vi "Parse Heatup Test Data.vi"(4 "34970 Data Raw":string[](array[string]), 5 "MW100 Data Raw":string[](array[string]), 6 "Agilent Read All?":bool=TRUE, 7 "Agilent Label Array":string[](array[string]), 8 "Serial Data":string="0:0:0 UE 36 LE 0 COMP 0 FAN1 0 FAN2 0 SP:0 0 0 0 0 0 C030", 9 "34970 Data":string[](array[string]), 10 "Power Data":string[](array[string]), 11 "MW100 Data":string[](array[string])) -> (2 "Output Data":string[][](array[string]))   [LabVIEW 2012]
uses:
  Global HEWH.vi
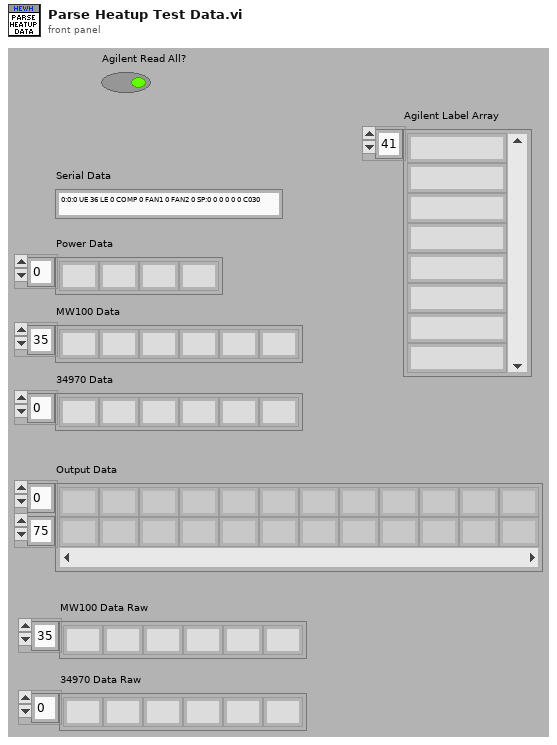
[diagram p1: front panel]
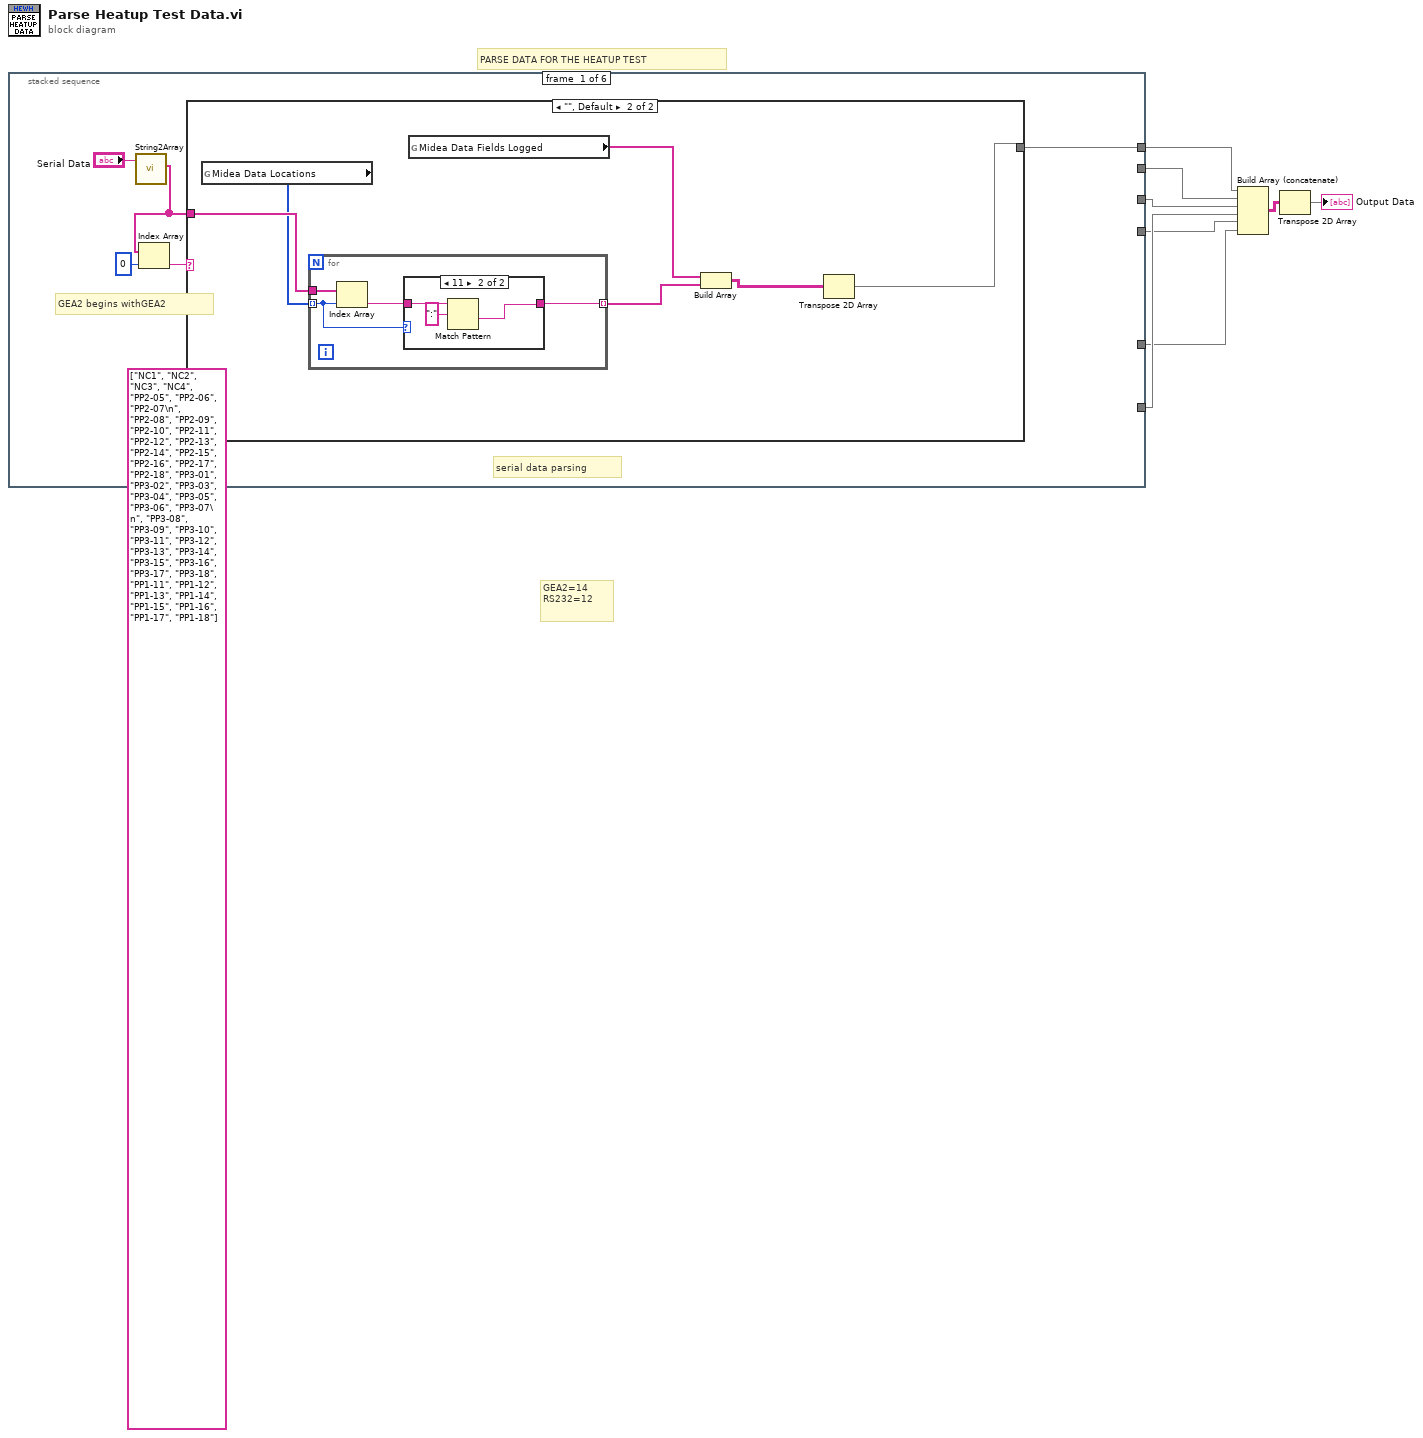
[diagram p0: block diagram]
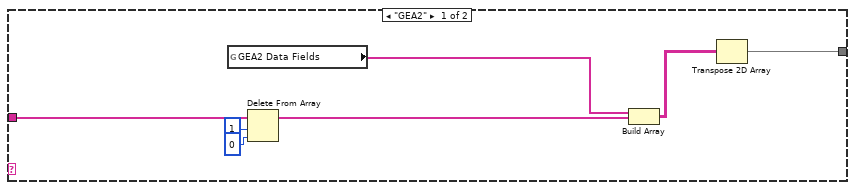
[diagram p2: hidden frame]
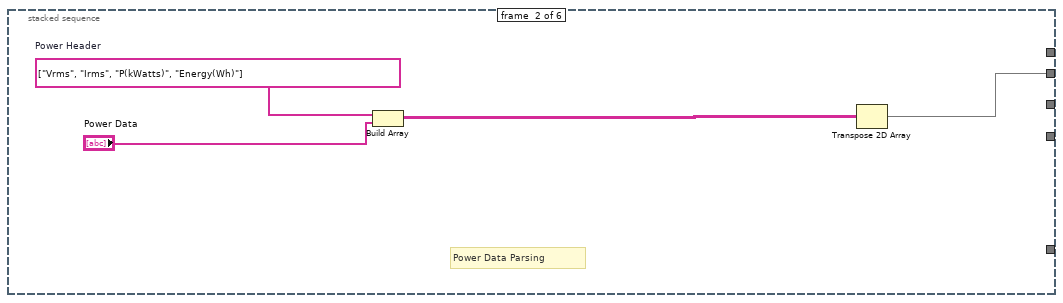
[diagram p4: hidden frame]
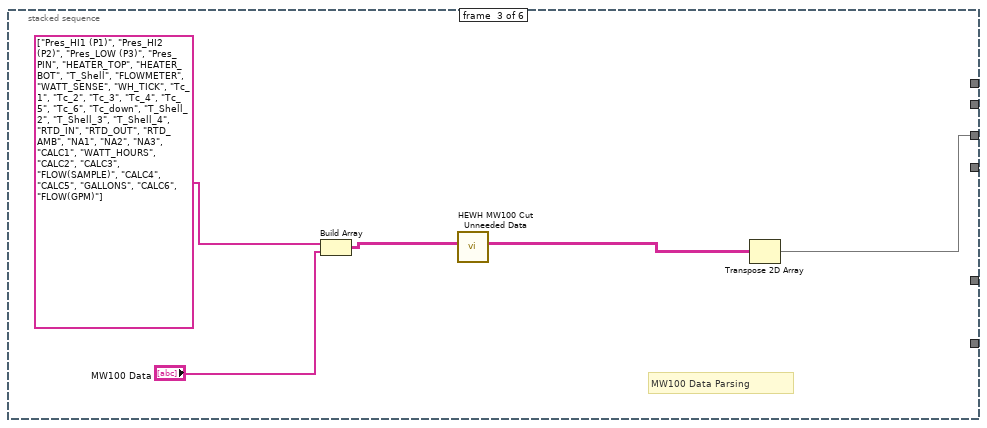
[diagram p5: hidden frame]
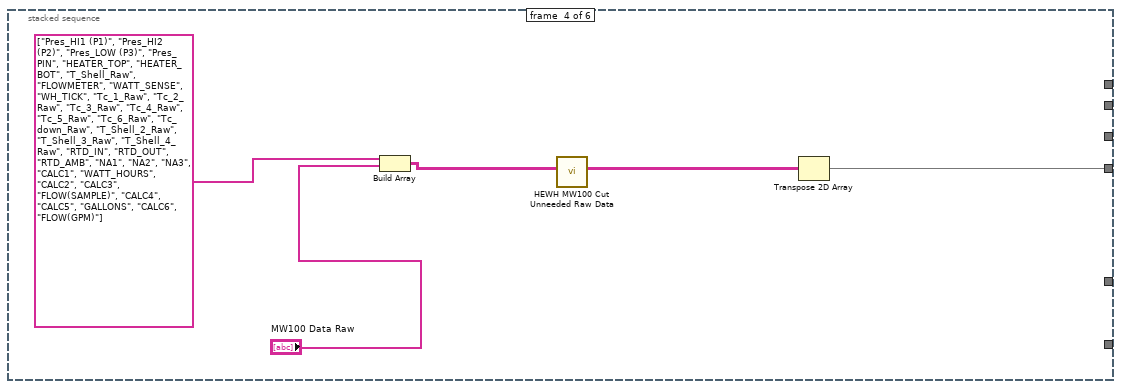
[diagram p6: hidden frame]
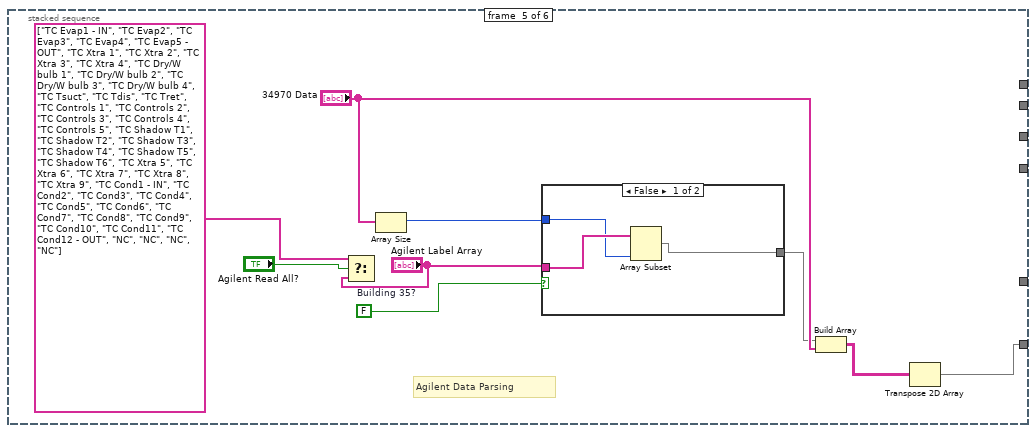
[diagram p7: hidden frame]
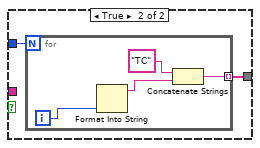
[diagram p8: hidden frame]
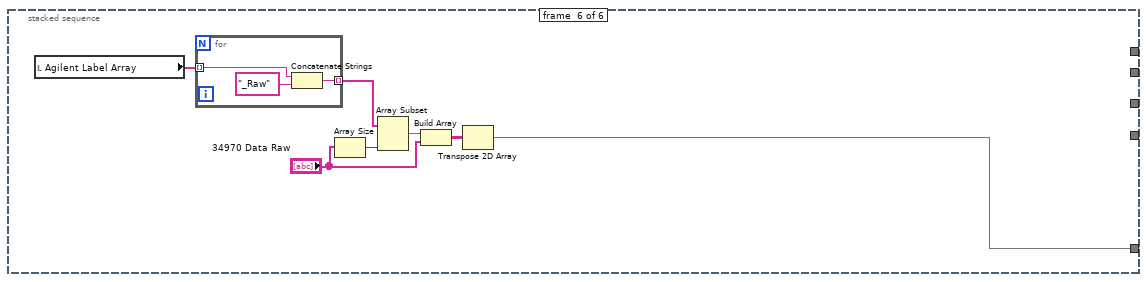
[diagram p9: hidden frame]
diagram:
  (unwired) string[] ["NC1", "NC2", "NC3", "NC4", "PP2-05", "PP2-06", "PP2-07\n", "PP2-08", "PP2-09", "PP2-10", "PP2-11", "PP2-12", "PP2-13", "PP2-14", "PP2-15", "PP2-16", "PP2-17", "PP2-18", "PP3-01", "PP3-02", "PP3-03", "PP3-04", "PP3-05", "PP3-06", "PP3-07\n", "PP3-08", "PP3-09", "PP3-10", "PP3-11", "PP3-12", "PP3-13", "PP3-14", "PP3-15", "PP3-16", "PP3-17", "PP3-18", "PP1-11", "PP1-12", "PP1-13", "PP1-14", "PP1-15", "PP1-16", "PP1-17", "PP1-18"] ("appended array")
  # "GEA2=14\nRS232=12"
  # "PARSE DATA FOR THE HEATUP TEST"
  n1 = stacked-sequence {
    tunnel: [w9 _ _ _ _ _] -> w7
    tunnel: [_ w35 _ _ _ _] -> w6
    tunnel: [_ _ w41 _ _ _] -> w4
    tunnel: [_ _ _ _ w50 _] -> w3
    tunnel: [_ _ _ w44 _ _] -> w2
    tunnel: [_ _ _ _ _ w67] -> w1
    frame #0 {
      # "GEA2 begins withGEA2"
      # "serial data parsing"
      n2 = call "String2Array.vi"("String"="Serial Data") -> ("Array"=w10:string[])  [unwired: 10 in]
      n3 = Index Array(array=w10, index=0) -> (element=w11:string)
      n4 = case shown="\"\", Default" w11 {
        tunnel: w10 -> [w18 w26]
        tunnel: [w19 w23] -> w9
        frame "GEA2" {
          n5 = global read "Global HEWH.vi" "GEA2 Data Fields"() -> (w14:string[])
          n6 = Delete From Array(array=w18, length=1, index=0) -> (array with subset deleted=w15:string[])  [unwired: 1 out]
          n7 = Build Array(w14, w15) -> (w20:string[][])
          n8 = Transpose 2D Array(2D array=w20) -> (transposed array=w19:string[][])
        }
        frame "", Default {
          n9 = global read "Global HEWH.vi" "Midea Data Locations"() -> (w21:i32[])
          n10 = for {
            tunnel: w26 -> [w30]
            tunnel: w21 -> [w29] mode=indexing
            tunnel: [w27] -> w25 mode=indexing
            n11 = Index Array(array=w30, index=w29) -> (element=w28:string)
            n12 = case shown="11" w29 {
              tunnel: w28 -> [w31 w34]
              tunnel: [w31 w32] -> w27
              frame 0, Default {
              }
              frame 11 {
                n13 = Match Pattern(string=w34, regular expression=":") -> (after substring=w32:string)  [unwired: 1 in, 3 out]
              }
            }
          }
          n14 = global read "Global HEWH.vi" "Midea Data Fields Logged"() -> (w22:string[])
          n15 = Build Array(w22, w25) -> (w24:string[][])
          n16 = Transpose 2D Array(2D array=w24) -> (transposed array=w23:string[][])
        }
      }
    }
    frame #1 {
      w36 = string[] ["Vrms", "Irms", "P(kWatts)", "Energy(Wh)"]  # Power Header
      # "Power Data Parsing"
      n17 = Build Array(w36, "Power Data") -> (w38:string[][])
      n18 = Transpose 2D Array(2D array=w38) -> (transposed array=w35:string[][])
    }
    frame #2 {
      # "MW100 Data Parsing"
      n19 = Build Array(string[] ["Pres_HI1 (P1)", "Pres_HI2 (P2)", "Pres_LOW (P3)", "Pres_PIN", "HEATER_TOP", "HEATER_BOT", "T_Shell", "FLOWMETER", "WATT_SENSE", "WH_TICK", "Tc_1", "Tc_2", "Tc_3", "Tc_4", "Tc_5", "Tc_6", "Tc_down", "T_Shell_2", "T_Shell_3", "T_Shell_4", "RTD_IN", "RTD_OUT", "RTD_AMB", "NA1", "NA2", "NA3", "CALC1", "WATT_HOURS", "CALC2", "CALC3", "FLOW(SAMPLE)", "CALC4", "CALC5", "GALLONS", "CALC6", "FLOW(GPM)"] ("output array"), "MW100 Data") -> (w40:string[][])
      n20 = call "HEWH MW100 Cut Unneeded Data.vi"("MW100 Data In"=w40) -> ("MW100 Data Out"=w39:string[][])  [unwired: 10 in]
      n21 = Transpose 2D Array(2D array=w39) -> (transposed array=w41:string[][])
    }
    frame #3 {
      n22 = Build Array(string[] ["Pres_HI1 (P1)", "Pres_HI2 (P2)", "Pres_LOW (P3)", "Pres_PIN", "HEATER_TOP", "HEATER_BOT", "T_Shell_Raw", "FLOWMETER", "WATT_SENSE", "WH_TICK", "Tc_1_Raw", "Tc_2_Raw", "Tc_3_Raw", "Tc_4_Raw", "Tc_5_Raw", "Tc_6_Raw", "Tc_down_Raw", "T_Shell_2_Raw", "T_Shell_3_Raw", "T_Shell_4_Raw", "RTD_IN", "RTD_OUT", "RTD_AMB", "NA1", "NA2", "NA3", "CALC1", "WATT_HOURS", "CALC2", "CALC3", "FLOW(SAMPLE)", "CALC4", "CALC5", "GALLONS", "CALC6", "FLOW(GPM)"] ("output array"), "MW100 Data Raw") -> (w46:string[][])
      n23 = call "HEWH MW100 Cut Unneeded Raw Data.vi"("MW100 Data In"=w46) -> ("MW100 Data Out"=w45:string[][])  [unwired: 10 in]
      n24 = Transpose 2D Array(2D array=w45) -> (transposed array=w44:string[][])
    }
    frame #4 {
      w56 = FALSE  # Building 35?
      # "Agilent Data Parsing"
      n25 = Select(t=string[] ["TC Evap1 - IN", "TC Evap2", "TC Evap3", "TC Evap4", "TC Evap5 - OUT", "TC Xtra 1", "TC Xtra 2", "TC Xtra 3", "TC Xtra 4", "TC Dry/W bulb 1", "TC Dry/W bulb 2", "TC Dry/W bulb 3", "TC Dry/W bulb 4", "TC Tsuct", "TC Tdis", "TC Tret", "TC Controls 1", "TC Controls 2", "TC Controls 3", "TC Controls 4", "TC Controls 5", "TC Shadow T1", "TC Shadow T2", "TC Shadow T3", "TC Shadow T4", "TC Shadow T5", "TC Shadow T6", "TC Xtra 5", "TC Xtra 6", "TC Xtra 7", "TC Xtra 8", "TC Xtra 9", "TC Cond1 - IN", "TC Cond2", "TC Cond3", "TC Cond4", "TC Cond5", "TC Cond6", "TC Cond7", "TC Cond8", "TC Cond9", "TC Cond10", "TC Cond11", "TC Cond12 - OUT", "NC", "NC", "NC", "NC"] ("output array"), s="Agilent Read All?", f="Agilent Label Array") -> ()  [unwired: 1 out]
      n26 = Array Size(array="34970 Data") -> (size(s)=w55:i32)
      n27 = case shown="False" w56 {
        tunnel: w55 -> [w59 w62]
        tunnel: [w58 w61] -> w53
        tunnel: "Agilent Label Array" -> [w60 _]
        frame False {
          n28 = Array Subset(array=w60, length=w59) -> (w58:string[])  [unwired: 1 in]
        }
        frame True {
          n29 = for {
            N: w62 -> [_]
            tunnel: [w63] -> w61 mode=indexing
            i -> [w66]
            n30 = Format Into String(w66) -> (resulting string=w65:string)  [unwired: 3 in, 1 out]
            n31 = Concatenate Strings("TC" ("string"), w65) -> (w63:string)
          }
        }
      }
      n32 = Build Array(w53, "34970 Data") -> (w51:string[][])
      n33 = Transpose 2D Array(2D array=w51) -> (transposed array=w50:string[][])
    }
    frame #5 {
      n34 = local read "Agilent Label Array"() -> (w69:string[])
      n35 = for {
        tunnel: w69 -> [w76] mode=indexing
        tunnel: [w74] -> w68 mode=indexing
        n36 = Concatenate Strings(w76, "_Raw" ("string")) -> (w74:string)
      }
      n37 = Array Size(array="34970 Data Raw") -> (size(s)=w73:i32)
      n38 = Array Subset(array=w68, length=w73) -> (w72:string[])  [unwired: 1 in]
      n39 = Build Array(w72, "34970 Data Raw") -> (w70:string[][])
      n40 = Transpose 2D Array(2D array=w70) -> (transposed array=w67:string[][])
    }
  }
  n41 = Build Array (concatenate)(w7, w6, w4, w3, w2, w1) -> (w8:string[][])
  n42 = Transpose 2D Array(2D array=w8) -> (transposed array=→"Output Data":string[][])
